vi "niRFUtil ERR Modify Errors.vi"(1 "Error codes":i32[](array[numeric]), 7 "error in (no error)":errorcluster, 12 "Modified Error\\Warning Codes":i32[](array[numeric]), 13 "Modified Error Source":string[](array[string])) -> (8 "error out":errorcluster)   [LabVIEW 2015, in "niRFUtil.lvlib"]
uses:
  niRFUtil.lvlib
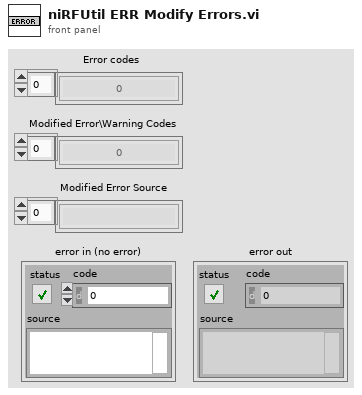
[diagram p1: front panel]
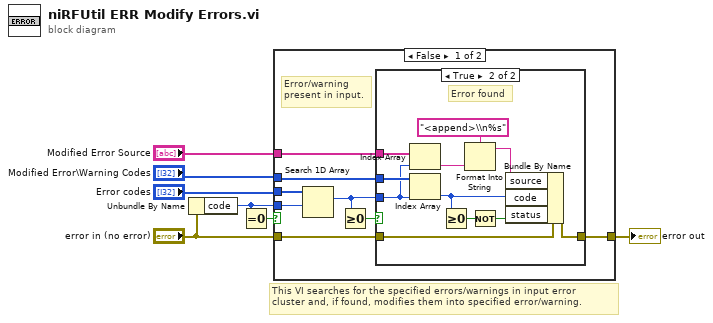
[diagram p0: block diagram]
diagram:
  # "This VI searches for the specified errors/warnings in input error \ncluster and, if found, modifies them into specified error/warning."
  n1 = Unbundle By Name("error in (no error)") -> ("code"=w1:i32)
  n2 = Equal To 0?(x=w1) -> (x = 0?=w2:bool)
  n3 = case shown="False" w2 {
    tunnel: [w13 w28] -> w7
    tunnel: "Error codes" -> [w15 _]
    tunnel: "Modified Error\\Warning Codes" -> [w9 _]
    tunnel: "Modified Error Source" -> [w10 _]
    tunnel: "error in (no error)" -> [w12 w28]
    tunnel: w1 -> [w11 _]
    frame False {
      # "Error/warning\npresent in input."
      n4 = Search 1D Array(1D array=w15, element=w11) -> (index of element=w8:i32)  [unwired: 1 in]
      n5 = Greater Or Equal To 0?(x=w8) -> (x >= 0?=w14:bool)
      n6 = case shown="True" w14 {
        tunnel: w12 -> [w16 w27]
        tunnel: [w16 w26] -> w13
        tunnel: w10 -> [_ w21]
        tunnel: w9 -> [_ w20]
        tunnel: w8 -> [_ w19]
        frame False {
          # "Error not found"
        }
        frame True {
          # "Error found"
          n7 = Index Array(array=w21, index=w19) -> (element=w18:string)
          n8 = Index Array(array=w20, index=w19) -> (element=w17:i32)
          n9 = Greater Or Equal To 0?(x=w17) -> (x >= 0?=w25:bool)
          n10 = Format Into String(format string="<append>\\n%s" ("source"), w18) -> (resulting string=w22:string)  [unwired: 2 in, 1 out]
          n11 = Not(x=w25) -> (.not. x?=w24:bool)
          n12 = Bundle By Name(cluster=w27, "source"=w22, "code"=w17, "status"=w24) -> (w26:errorcluster)
        }
      }
    }
    frame True {
      # "No error/warning"
    }
  }
  "error out" <- w7
